vi "GUI Interlocks.vi"(10 "Power State":bool, 11 "References":T1) -> ()   [LabVIEW 2015, in "Device Under Test_Cloneable_DQMH.lvlib"]
doc: "This VI determines if the Power On, Power Off and Self Test Buttons are enabled or disabled depending on the current power state.\n____\nDelacor QMH Thermal Chamber Examples 4.0.0.21\nCopyright (c) 2018, Delacor"
uses:
  Device Under Test_Cloneable_DQMH.lvlib
  GUI Control References--cluster.ctl
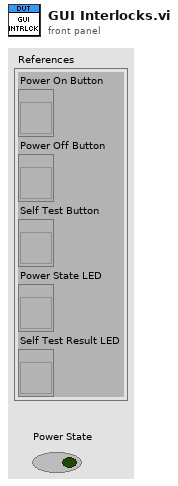
[diagram p1: front panel]
types:
  T1 = typedef "Device Under Test_Cloneable_DQMH.lvlib/GUI Control References--cluster.ctl" = cluster{"Power On Button":refnum<vi>, "Power Off Button":refnum<vi>, "Self Test Button":refnum<vi>, "Power State LED":refnum<vi>, "Self Test Result LED":refnum<vi>}
  T2 = enum8{"Enabled", "Disabled", "Disabled and Grayed Out"}
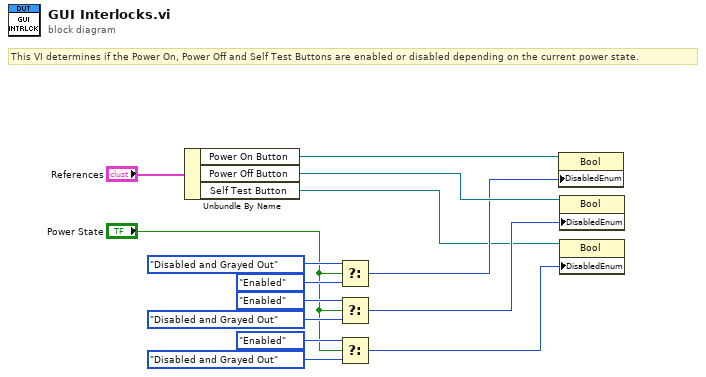
[diagram p0: block diagram]
diagram:
  # "This VI determines if the Power On, Power Off and Self Test Buttons are enabled or disabled depending on the current power state."
  n1 = Unbundle By Name("References") -> ("Power On Button"=w1:refnum<vi>, "Power Off Button"=w8:refnum<vi>, "Self Test Button"=w4:refnum<vi>)
  n2 = Select(t=T2."Disabled and Grayed Out" ("Disabled"), s="Power State", f=T2."Enabled" ("Disabled")) -> (s? t:f=w7:T2)
  n3 = Select(t=T2."Enabled" ("Disabled"), s="Power State", f=T2."Disabled and Grayed Out" ("Disabled")) -> (s? t:f=w6:T2)
  n4 = Select(t=T2."Enabled" ("Disabled"), s="Power State", f=T2."Disabled and Grayed Out" ("Disabled")) -> (s? t:f=w5:T2)
  n5 = property class="Bool"(reference=w1, "DisabledEnum"=w7) -> ()  [unwired: 1 in, 2 out]
  n6 = property class="Bool"(reference=w8, "DisabledEnum"=w6) -> ()  [unwired: 1 in, 2 out]
  n7 = property class="Bool"(reference=w4, "DisabledEnum"=w5) -> ()  [unwired: 1 in, 2 out]
